vi "Latcher.vi"(5 "Value In":bool) -> (2 "Latched":bool)   [LabVIEW 2014]
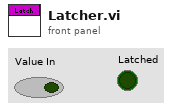
[diagram p1: front panel]
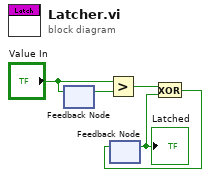
[diagram p0: block diagram]
diagram:
  n1 = feedback #1() -> (w3:bool)  [unwired: 1 in]
  n2 = feedback-in #1("Value In") -> ()
  n3 = Greater?(x="Value In", y=w3) -> (0:w1:bool)
  n4 = feedback #2() -> (w4:bool)  [unwired: 1 in]
  "Latched" <- w4
  n5 = Exclusive Or(1:w4, 2:w1) -> (0:w5:bool)
  n6 = feedback-in #2(w5) -> ()
